vi "DSF.Transceiver.UDP.Settings.Transfer Group.vi"(8 "error in (no error)":errorcluster, 10 "Transfer Groups Configurations":refnum<class "DSF.Shared.Configuration.Transfer Group.lvclass">[](array[class]), 11 "UDP Transceiver in":refnum<class "DSF.Transceiver.UDP.lvclass">) -> (0 "error out":errorcluster, 3 "UDP Transceiver out":refnum<class "DSF.Transceiver.UDP.lvclass">)   [LabVIEW 2017, in "DSF.Transceiver.UDP.lvlib" / "DSF.Transceiver.UDP.lvclass"]
uses:
  DSF.Transceiver.UDP.lvclass
  DSF Core/Built/Engine/DSF.Engine.lvlibp/Shared/Classes/Transfer Group/DSF.Shared.Configuration.Transfer Group.lvclass
  DSF.Transceiver.UDP.lvclass/DSF.Transceiver.UDP.ctl
  DSF.Transceiver.UDP.Parameters.Transfer Group.ctl
  DSF.Transceiver.UDP.Parameters.Transfer Group.Rx.ctl
  DSF.Transceiver.UDP.Parameters.Transfer.Rx.ctl
  DSF.Transceiver.UDP.Parameters.Transfer Group.Tx.ctl
  DSF.Transceiver.UDP.Parameters.Transfer.Tx.ctl
  DSF Core/Built/Engine/DSF.Engine.lvlibp/Shared/Classes/Configuration/DSF.Shared.Configuration.lvclass
  DSF Core/Built/Engine/DSF.Engine.lvlibp/Shared/Classes/Transfer/DSF.Shared.Configuration.Transfer.lvclass
  C:/Git/DSF/DSF Core/Built/Engine/DSF.Engine.lvlibp/Shared/Classes/Configuration/DSF.Shared.Configuration.lvclass
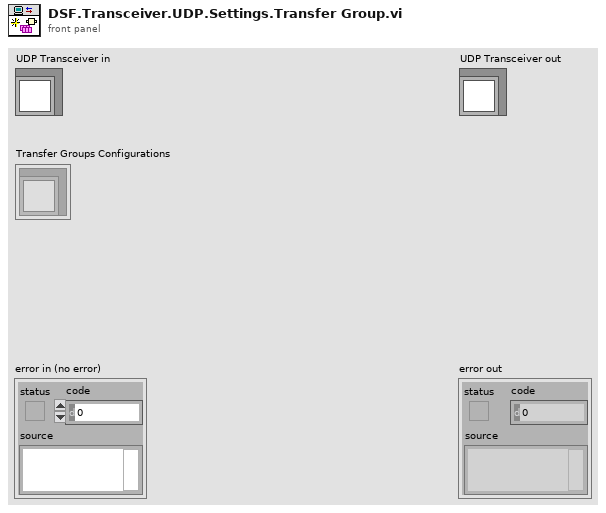
[diagram p1: front panel]
types:
  T1 = typedef "DSF.Transceiver.UDP.lvlib/DSF.Transceiver.UDP.lvclass/DSF.Transceiver.UDP.Parameters.Transfer Group.ctl" = cluster{"Rx":T2, "Tx":T4}
  T2 = typedef "DSF.Transceiver.UDP.lvlib/DSF.Transceiver.UDP.lvclass/DSF.Transceiver.UDP.Parameters.Transfer Group.Rx.ctl" = cluster{"Transfers Rx":T3[], "max size":i32}
  T3 = typedef "DSF.Transceiver.UDP.lvlib/DSF.Transceiver.UDP.lvclass/DSF.Transceiver.UDP.Parameters.Transfer.Rx.ctl" = cluster{"timeout":i32, "source address":u32, "source port":u16}
  T4 = typedef "DSF.Transceiver.UDP.lvlib/DSF.Transceiver.UDP.lvclass/DSF.Transceiver.UDP.Parameters.Transfer Group.Tx.ctl" = cluster{"Transfers Tx":T5[]}
  T5 = typedef "DSF.Transceiver.UDP.lvlib/DSF.Transceiver.UDP.lvclass/DSF.Transceiver.UDP.Parameters.Transfer.Tx.ctl" = cluster{"destination port":u16, "destination address":u32}
  T6 = typedef "DSF.Engine.lvlibp/DSF Configuration API.lvlib/DSF Direction.ctl" = enum8{"Tx", "Rx"}
  T7 = typedef "DSF.Engine.lvlibp/DSF Configuration API.lvlib/DSF Settings Info.ctl" = cluster{"key":string, "value":string}[]
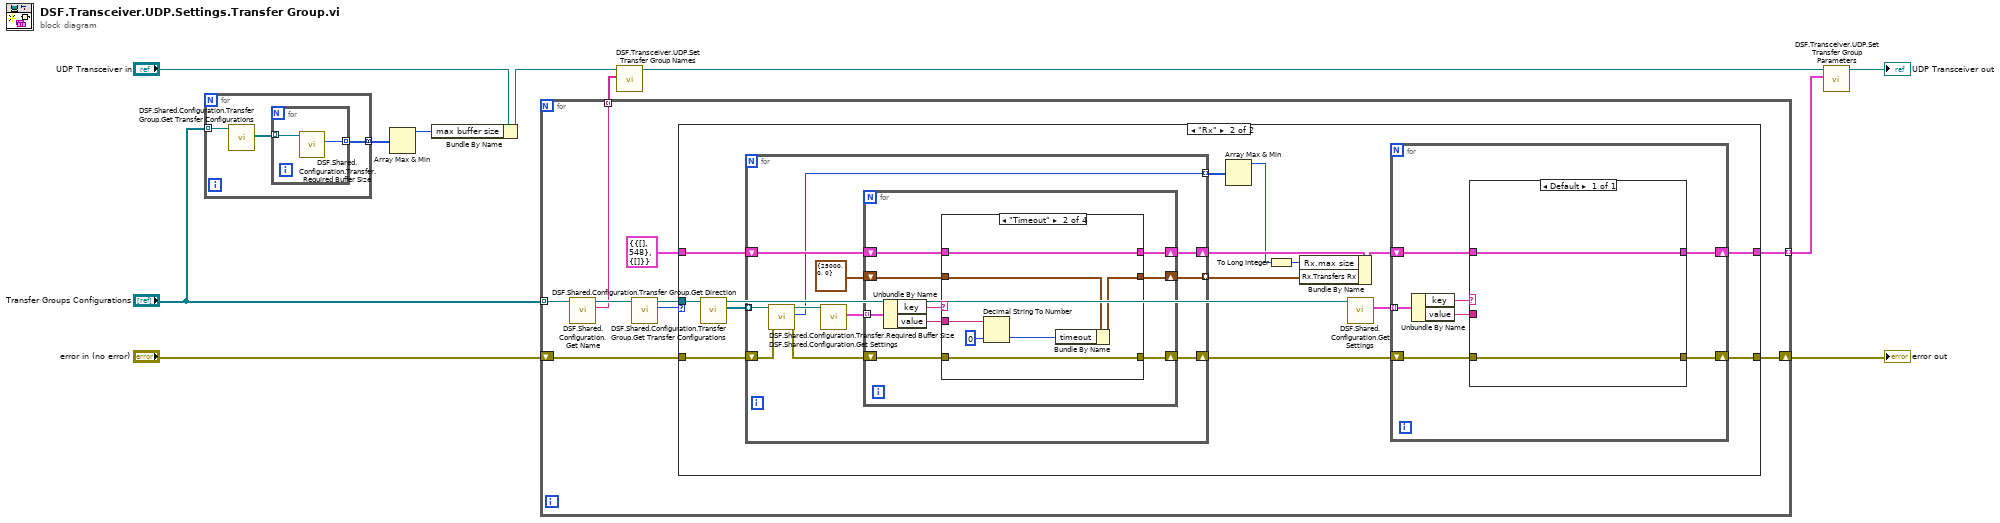
[diagram p0: block diagram]
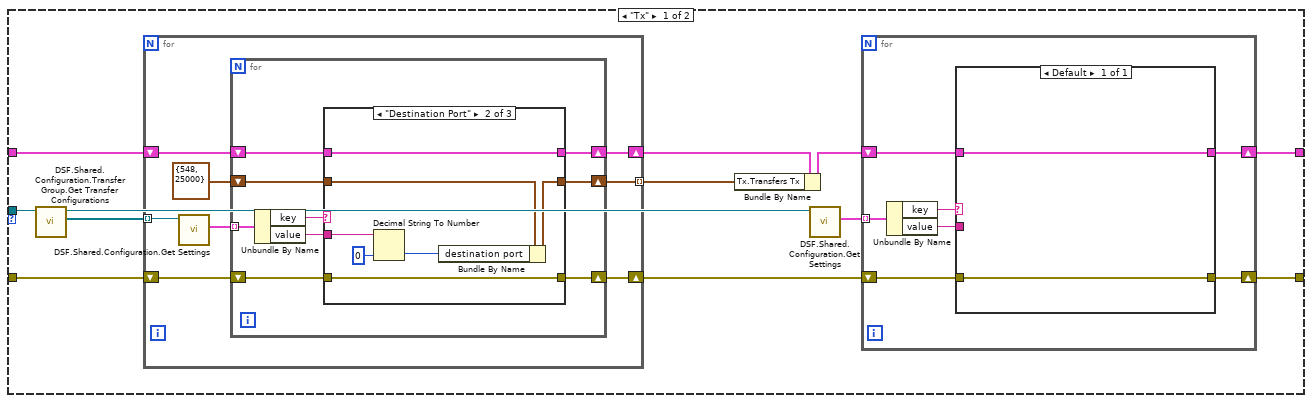
[diagram p2: hidden frame]
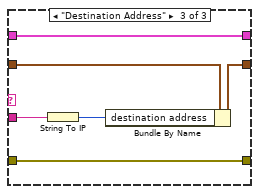
[diagram p4: hidden frame]
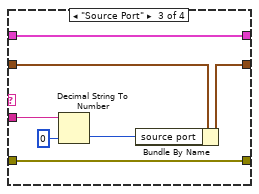
[diagram p6: hidden frame]
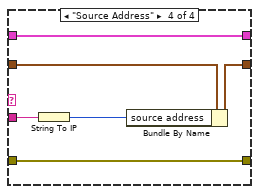
[diagram p7: hidden frame]
diagram:
  n1 = for {
    tunnel: "Transfer Groups Configurations" -> [w14] mode=indexing
    tunnel: [w12] -> w8 mode=concatenating
    n2 = call "DSF.Shared.Configuration.Transfer Group.Get Transfer Configurations.vi"("Transfer Group Configuration in"=w14) -> ("Transfer Configurations"=w13:refnum<class "DSF.Shared.Configuration.Transfer.lvclass">[])  [unwired: 9 in, 1 out]
    n3 = for {
      tunnel: w13 -> [w16] mode=indexing
      tunnel: [w15] -> w12 mode=indexing
      n4 = call "DSF.Shared.Configuration.Transfer.Required Buffer Size.vi"("Transfer Configuration in"=w16) -> ("required buffer size"=w15:u64)  [unwired: 8 in, 2 out]
    }
  }
  n5 = Array Max & Min(array=w8) -> (max value=w6:u64)  [unwired: 3 out]
  n6 = Bundle By Name(cluster="UDP Transceiver in", "max buffer size"=w6) -> (w4:refnum<class "DSF.Transceiver.UDP.lvclass">)
  n7 = for {
    tunnel: "Transfer Groups Configurations" -> [w17] mode=indexing
    tunnel: [w24] -> w9 mode=indexing
    tunnel: [w21] -> w2 mode=indexing
    shift-right: [w19] -> w10
    shift-left: "error in (no error)" -> [w20]
    n8 = call "DSF.Shared.Configuration.Get Name.vi"("Configuration in"=w17) -> ("name"=w24:string, "Configuration out"=w25:refnum<class "DSF.Shared.Configuration.Transfer Group.lvclass">)  [unwired: 9 in]
    n9 = call "DSF.Shared.Configuration.Transfer Group.Get Direction.vi"("Transfer Group Configuration in"=w25) -> ("direction"=w22:T6, "Transfer Group Configuration out"=w23:refnum<class "DSF.Shared.Configuration.Transfer Group.lvclass">)  [unwired: 9 in]
    n10 = case shown="\"Rx\"" w22 {
      tunnel: w23 -> [w31 w86]
      tunnel: T1 {"Rx"={"Transfers Rx"=[], "max size"=548}, "Tx"={"Transfers Tx"=[]}} ("Rx/Tx Parameters") -> [w32 w87]
      tunnel: [w36 w94] -> w21
      tunnel: w20 -> [w34 w88]
      tunnel: [w35 w93] -> w19
      frame "Tx" {
        n11 = call "DSF.Shared.Configuration.Transfer Group.Get Transfer Configurations.vi"("Transfer Group Configuration in"=w31) -> ("Transfer Configurations"=w29:refnum<class "DSF.Shared.Configuration.Transfer.lvclass">[], "Transfer Group Configuration out"=w30:refnum<class "DSF.Shared.Configuration.Transfer Group.lvclass">)  [unwired: 9 in]
        n12 = for {
          shift-right: [w44] -> w28
          shift-left: w32 -> [w45]
          shift-right: [w42] -> w33
          shift-left: w34 -> [w43]
          tunnel: w29 -> [w41] mode=indexing
          tunnel: [w38] -> w27 mode=indexing
          n13 = call "DSF.Shared.Configuration.Get Settings.vi"("Configuration in"=w41) -> ("settings"=w40:T7)  [unwired: 9 in, 1 out]
          n14 = for {
            tunnel: w40 -> [w48] mode=indexing
            shift-right: [w51] -> w44
            shift-left: w45 -> [w52]
            shift-right: [w49] -> w42
            shift-left: w43 -> [w50]
            shift-right: [w47] -> w38
            shift-left: T5 {"destination port"=548, "destination address"=25000} ("Transfer Tx") -> [w46]
            n15 = Unbundle By Name(w48) -> ("key"=w54:string, "value"=w53:string)
            n16 = case shown="\"Destination Port\"" w54 {
              tunnel: w53 -> [_ w64 w69]
              tunnel: w52 -> [w57 w59 w66]
              tunnel: [w57 w59 w66] -> w51
              tunnel: w50 -> [w56 w61 w70]
              tunnel: [w56 w61 w70] -> w49
              tunnel: w46 -> [w55 w60 w67]
              tunnel: [w55 w58 w65] -> w47
              frame Default {
              }
              frame "Destination Port" {
                n17 = Decimal String To Number(string=w64, default (0L)=u16 0 ("default (0 I32)")) -> (number=w62:u16)  [unwired: 1 in, 1 out]
                n18 = Bundle By Name(cluster=w60, "destination port"=w62) -> (w58:T5)
              }
              frame "Destination Address" {
                n19 = String To IP(1:w69) -> (0:w68:u32)
                n20 = Bundle By Name(cluster=w67, "destination address"=w68) -> (w65:T5)
              }
            }
          }
        }
        n21 = Bundle By Name(cluster=w28, "Tx.Transfers Tx"=w27) -> (w26:T1)
        n22 = call "DSF.Shared.Configuration.Get Settings.vi"("Configuration in"=w30) -> ("settings"=w37:T7)  [unwired: 9 in, 1 out]
        n23 = for {
          tunnel: w37 -> [w75] mode=indexing
          shift-right: [w73] -> w36
          shift-left: w26 -> [w74]
          shift-right: [w71] -> w35
          shift-left: w33 -> [w72]
          n24 = Unbundle By Name(w75) -> ("key"=w77:string, "value"=w76:string)
          n25 = case shown="Default" w77 {
            tunnel: w76 -> [_]
            tunnel: w74 -> [w79]
            tunnel: [w79] -> w73
            tunnel: w72 -> [w78]
            tunnel: [w78] -> w71
            frame Default {
            }
          }
        }
      }
      frame "Rx" {
        n26 = call "DSF.Shared.Configuration.Transfer Group.Get Transfer Configurations.vi"("Transfer Group Configuration in"=w86) -> ("Transfer Configurations"=w91:refnum<class "DSF.Shared.Configuration.Transfer.lvclass">[], "Transfer Group Configuration out"=w92:refnum<class "DSF.Shared.Configuration.Transfer Group.lvclass">)  [unwired: 9 in]
        n27 = for {
          shift-right: [w104] -> w90
          shift-left: w87 -> [w105]
          shift-right: [w103] -> w83
          shift-left: w88 -> [w97]
          tunnel: w91 -> [w99] mode=indexing
          tunnel: [w100] -> w89 mode=indexing
          tunnel: [w95] -> w82 mode=indexing
          n28 = call "DSF.Shared.Configuration.Transfer.Required Buffer Size.vi"("error in (no error)"=w97, "Transfer Configuration in"=w99) -> ("error out"=w96:errorcluster, "required buffer size"=w95:u64, "Transfer Configuration out"=w98:refnum<class "DSF.Shared.Configuration.Transfer.lvclass">)  [unwired: 7 in]
          n29 = call "DSF.Shared.Configuration.Get Settings.vi"("Configuration in"=w98) -> ("settings"=w102:T7)  [unwired: 9 in, 1 out]
          n30 = for {
            tunnel: w102 -> [w108] mode=indexing
            shift-right: [w111] -> w104
            shift-left: w105 -> [w112]
            shift-right: [w109] -> w103
            shift-left: w96 -> [w110]
            shift-right: [w107] -> w100
            shift-left: T3 {"timeout"=25000, "source address"=0, "source port"=0} ("Transfer Rx") -> [w106]
            n31 = Unbundle By Name(w108) -> ("key"=w114:string, "value"=w113:string)
            n32 = case shown="\"Timeout\"" w114 {
              tunnel: w113 -> [_ w124 w131 w133]
              tunnel: w112 -> [w117 w119 w126 w135]
              tunnel: [w117 w119 w126 w135] -> w111
              tunnel: w110 -> [w116 w121 w128 w137]
              tunnel: [w116 w121 w128 w137] -> w109
              tunnel: w106 -> [w115 w120 w127 w136]
              tunnel: [w115 w118 w125 w134] -> w107
              frame Default {
              }
              frame "Timeout" {
                n33 = Decimal String To Number(string=w124, default (0L)=0 ("default (0 I32)")) -> (number=w122:i32)  [unwired: 1 in, 1 out]
                n34 = Bundle By Name(cluster=w120, "timeout"=w122) -> (w118:T3)
              }
              frame "Source Port" {
                n35 = Decimal String To Number(string=w131, default (0L)=u16 0 ("default (0 I32)")) -> (number=w129:u16)  [unwired: 1 in, 1 out]
                n36 = Bundle By Name(cluster=w127, "source port"=w129) -> (w125:T3)
              }
              frame "Source Address" {
                n37 = String To IP(1:w133) -> (0:w132:u32)
                n38 = Bundle By Name(cluster=w136, "source address"=w132) -> (w134:T3)
              }
            }
          }
        }
        n39 = Array Max & Min(array=w82) -> (max value=w81:u64)  [unwired: 3 out]
        n40 = To Long Integer(number=w81) -> (32bit integer=w80:i32)
        n41 = Bundle By Name(cluster=w90, "Rx.max size"=w80, "Rx.Transfers Rx"=w89) -> (w85:T1)
        n42 = call "DSF.Shared.Configuration.Get Settings.vi"("Configuration in"=w92) -> ("settings"=w84:T7)  [unwired: 9 in, 1 out]
        n43 = for {
          tunnel: w84 -> [w142] mode=indexing
          shift-right: [w140] -> w94
          shift-left: w85 -> [w141]
          shift-right: [w138] -> w93
          shift-left: w83 -> [w139]
          n44 = Unbundle By Name(w142) -> ("key"=w144:string, "value"=w143:string)
          n45 = case shown="Default" w144 {
            tunnel: w143 -> [_]
            tunnel: w141 -> [w146]
            tunnel: [w146] -> w140
            tunnel: w139 -> [w145]
            tunnel: [w145] -> w138
            frame Default {
            }
          }
        }
      }
    }
  }
  "error out" <- w10
  n46 = call "DSF.Transceiver.UDP.Set Transfer Group Names.vi"("Transfer Group names"=w9, "UDP Transceiver in"=w4) -> ("UDP Transceiver out"=w3:refnum<class "DSF.Transceiver.UDP.lvclass">)  [unwired: 9 in]
  n47 = call "DSF.Transceiver.UDP.Set Transfer Group Parameters.vi"("Transfer Group parameters"=w2, "UDP Transceiver in"=w3) -> ("UDP Transceiver out"=→"UDP Transceiver out":refnum<class "DSF.Transceiver.UDP.lvclass">)  [unwired: 9 in]
